vi "CreateTask.vi"(2 "error in (no error)":errorcluster, 3 "Task path":string) -> (0 "error out":errorcluster, 1 "Task ID":u32)   [LabVIEW 2009]
doc: "Create task according to task file path."
uses:
  Windows/System32/AdvLvDaq.dll
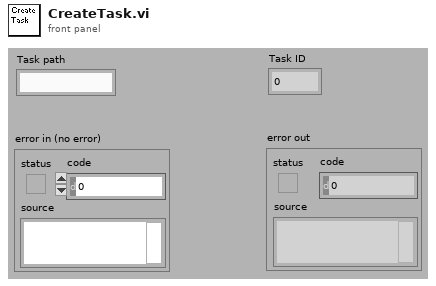
[diagram p1: front panel]
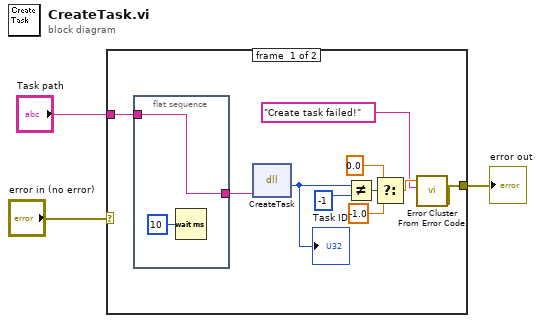
[diagram p0: block diagram]
diagram:
  n1 = case shown="No Error" "error in (no error)" {
    selector: "error in (no error)" -> [_ w16]
    tunnel: [w6 w16] -> w2
    tunnel: "Task path" -> [w4 _]
    frame #0 {
      n2 = flat-sequence {
        tunnel: [w15] -> w5
        tunnel: w4 -> [w15]
        frame #0 {
          n3 = Wait (ms)(milliseconds to wait=u32 10) -> ()  [unwired: 1 out]
        }
      }
      n4 = dll-call lib="C:/Windows/System32/AdvLvDaq.dll" fn="CreateTask"("taskPath"=w5) -> ("return type"=w12:i32)  [unwired: 4 in, 2 out]
      "Task ID" <- w12
      n5 = Not Equal?(x=w12, y=-1) -> (x != y?=w11:bool)
      n6 = Select(t=0.0, s=w11, f=-1.0) -> (s? t:f=w8:dbl)
      n7 = call <vilib>:"Error Cluster From Error Code.vi"("error message (\"\")"="Create task failed!" ("error message (\"\")"), "error code (0)"=w8) -> ("error out"=w6:errorcluster)  [unwired: 2 in, 5 out]
    }
    frame #1 {
    }
  }
  "error out" <- w2
